vi "SH_ComputeFitnessClassifier.vi"(8 "error in (no error)":errorcluster, 9 "Notifier":refnum<notifier>, 10 "Shapelets Queue":refnum<queue>, 11 "ShapeletClass in":refnum<class "Shapelets Search Brute Force.lvclass">) -> (0 "error out":errorcluster, 2 "Fitness Values":dbl[](array[numeric]), 3 "ShapeletClass out":refnum<class "Shapelets Search Brute Force.lvclass">)   [LabVIEW 2016, in "Shapelets Search (Brute Force).lvlib" / "Shapelets Search Brute Force.lvclass"]
uses:
  Shapelets Search Brute Force.lvclass
  SH_Shapelet.ctl
  Shapelets Search Brute Force.lvclass/Shapelets Search Brute Force.ctl
  <vilib>/Analysis/baseanly.llb/Normalize Vector.vi
  Shapelets Search (Brute Force).lvlib
  <vilib>/Analysis/NI_AALBase.lvlib
panel:
  # "This VI is a part of BCI Design library, http://www.ru-bci.org \nCopyright © 2020, Sotnikov Peter, All rights reserved. License: CC BY-NC 4.0"
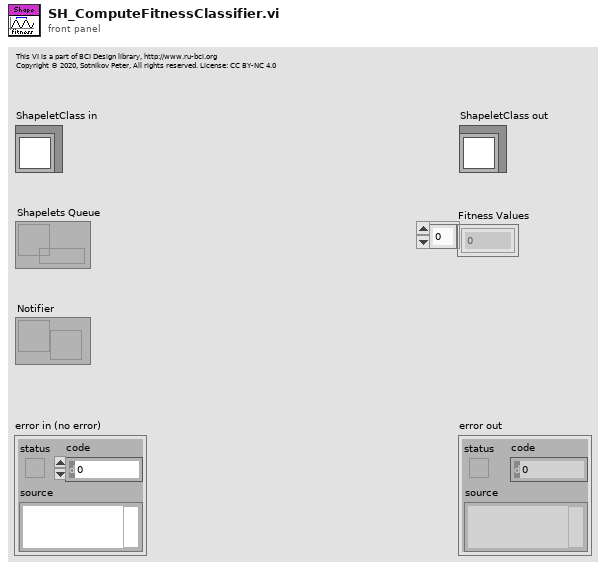
[diagram p1: front panel]
types:
  T1 = cluster{"ClassLabel":string, "FeatureVector":dbl[][]}[]
  T2 = typedef "Shapelets Search (Brute Force).lvlib/SH_Shapelet.ctl" = cluster{"TrialIndex":i32, "Shift (in samples)":i32, "Length (in samples)":i32, "Distances":dbl[], "ClassIndecies":i32[], "Fitness":dbl, "Split Point":dbl}
  T3 = cluster{"ClassLabel":string, "FeatureVector":dbl[][]}
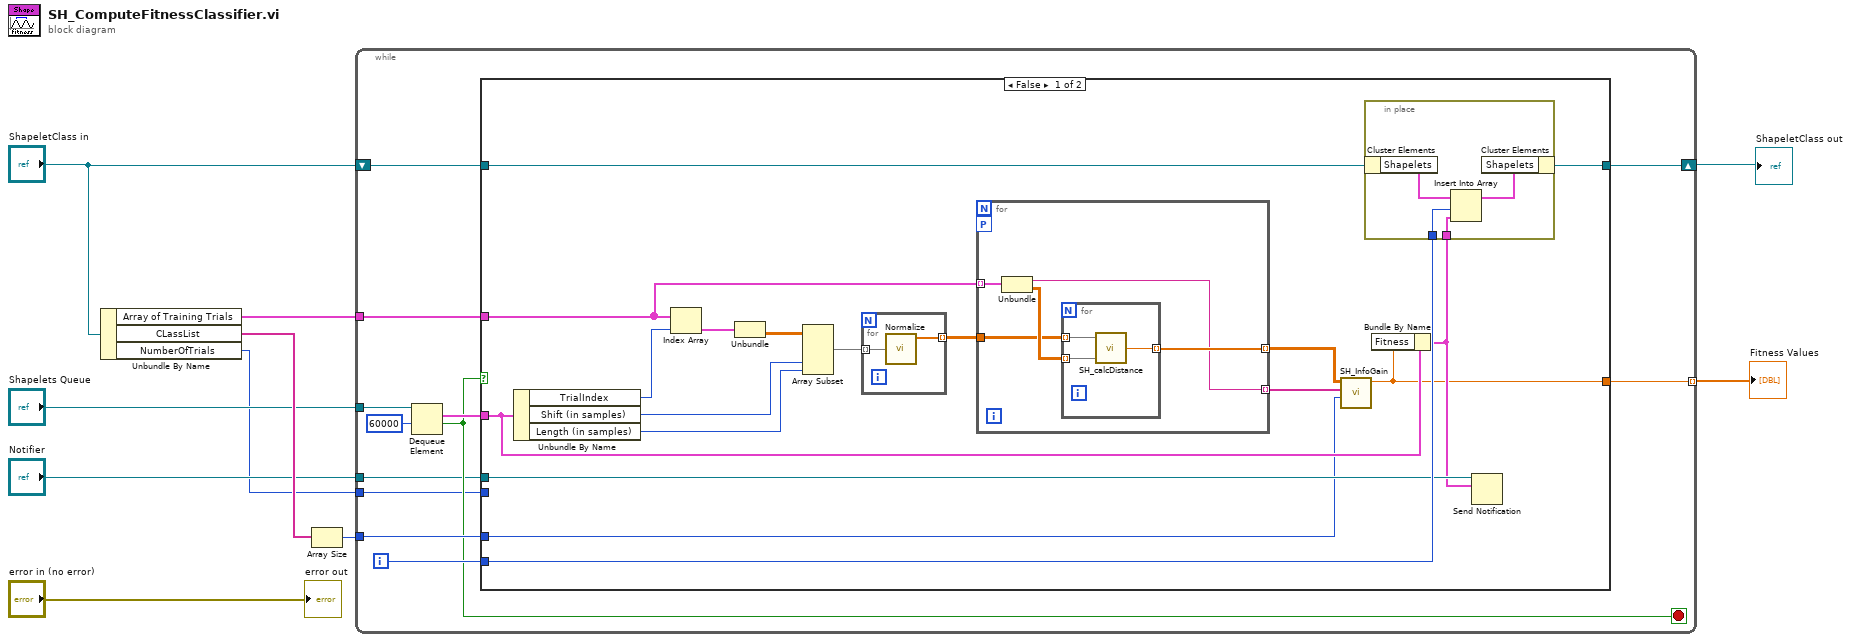
[diagram p0: block diagram]
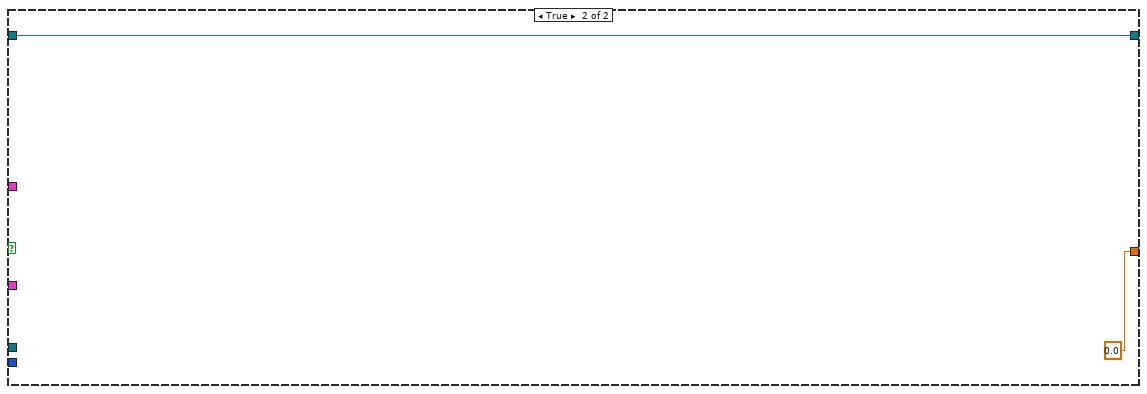
[diagram p2: hidden frame]
diagram:
  n1 = Unbundle By Name("ShapeletClass in") -> ("Array of Training Trials"=w10:T1, "CLassList"=w5:string[], "NumberOfTrials"=w1:i32)
  n2 = Array Size(array=w5) -> (size(s)=w6:i32)
  n3 = while {
    tunnel: w10 -> [w22]
    shift-right: [w20] -> w8
    shift-left: "ShapeletClass in" -> [w21]
    tunnel: w6 -> [w19]
    tunnel: [w17] -> w4 mode=indexing
    tunnel: "Shapelets Queue" -> [w16]
    tunnel: "Notifier" -> [w12]
    tunnel: w1 -> [w11]
    i -> [w18]
    stop <- w13 stop-if-true
    n4 = Dequeue Element(queue=w16, timeout in ms (-1)=60000) -> (element=w15:T2, timed out?=w13:bool)  [unwired: 1 in, 2 out]
    n5 = case shown="False" w13 {
      tunnel: w22 -> [w37 _]
      tunnel: w21 -> [w35 w56]
      tunnel: [w34 w56] -> w20
      tunnel: w19 -> [w24 _]
      tunnel: w18 -> [w33 _]
      tunnel: [w23 0.0 ("f")] -> w17
      tunnel: w15 -> [w32 _]
      tunnel: w12 -> [w31 _]
      tunnel: w11 -> [_ _]
      frame False {
        n6 = Unbundle By Name(w32) -> ("TrialIndex"=w40:i32, "Shift (in samples)"=w28:i32, "Length (in samples)"=w29:i32)
        n7 = Index Array(array=w37, index=w40) -> (element=w39:T3)
        n8 = Unbundle(w39) -> ("FeatureVector"=w38:dbl[][])  [unwired: 1 out]
        n9 = Array Subset(array=w38, index (col)=w28, length (col)=w29) -> (w27:dbl[][])  [unwired: 2 in]
        n10 = for {
          tunnel: [w42] -> w36 mode=indexing
          tunnel: w27 -> [w41] mode=indexing
          n11 = call-poly <vilib>:"Normalize.vi"("Vector"=w41) -> ("Normalized Vector"=w42:dbl[])  [unwired: 1 in, 3 out]
        }
        n12 = for {
          tunnel: w37 -> [w51] mode=indexing
          tunnel: w36 -> [w49]
          workers-P: _ -> [_]
          tunnel: [w48] -> w26 mode=indexing
          tunnel: [w47] -> w25 mode=indexing
          n13 = Unbundle(w51) -> ("ClassLabel"=w47:string, "FeatureVector"=w50:dbl[][])
          n14 = for {
            tunnel: w50 -> [w53] mode=indexing
            tunnel: w49 -> [w54] mode=indexing
            tunnel: [w52] -> w48 mode=indexing
            n15 = call "SH_calcDistance.vi"("Time series"=w53, "Shapelet (normalized)"=w54) -> ("Distance out"=w52:dbl)  [unwired: 1 in]
          }
        }
        n16 = call "SH_InfoGain.vi"("NumberOfClasses"=w24, "Class Labels"=w25, "Distancies"=w26) -> ("Accuracy"=w23:sgl)  [unwired: 7 in, 1 out]
        n17 = Bundle By Name(cluster=w32, "Fitness"=w23) -> (w30:T2)
        n18 = in-place {
          in-place-border: w33 -> [w44]
          in-place-border: w30 -> [w43]
          n19 = in-place-cluster #1(w35) -> ("Shapelets"=w46:T2[])
          n20 = Insert Into Array(array=w46, index=w44, new element=w43) -> (w45:T2[])
          n21 = in-place-cluster #1("Shapelets"=w45) -> (w34:refnum<class "Shapelets Search Brute Force.lvclass">)
        }
        n22 = Send Notification(notification=w30, notifier=w31) -> ()  [unwired: 1 in, 2 out]
      }
      frame True {
      }
    }
  }
  "ShapeletClass out" <- w8
  "Fitness Values" <- w4
  "error out" <- "error in (no error)"
